vi "Clear.vi"(8 "error in (no error)":errorcluster, 11 "PQ Result  in":refnum<class "PQ Result.lvclass">) -> (0 "error out":errorcluster)   [LabVIEW 2015, in "PQ Result.lvclass"]
doc: "Clears (frees resources) of a PG result set. This operates even on error in."
uses:
  PQ Result.lvclass
  PQ Result.lvclass/PQ Result.ctl
  Connection/libpq.dll
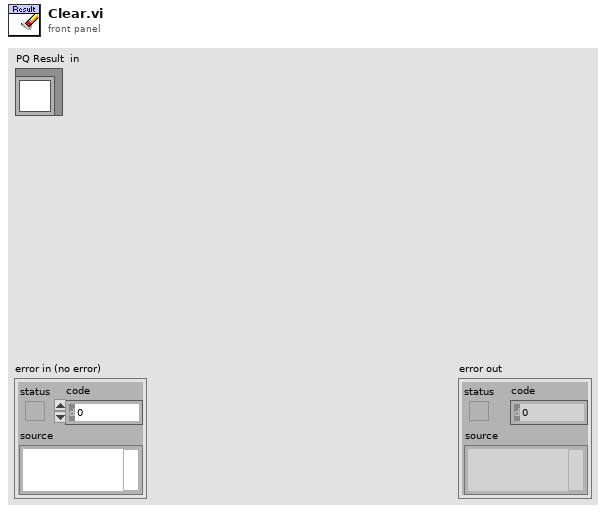
[diagram p1: front panel]
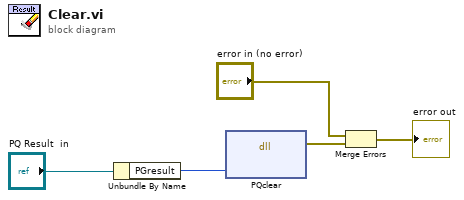
[diagram p0: block diagram]
diagram:
  n1 = Unbundle By Name("PQ Result  in") -> ("PGresult"=w2:u32)
  n2 = dll-call lib="C:/PQ/Connection/libpq.dll" fn="PQclear"("PGresult"=w2) -> (error out=w1:errorcluster)  [unwired: 5 in, 1 out]
  n3 = Merge Errors("error in (no error)", w1) -> (→"error out":errorcluster)
